vi "myRIO_BRig_RT__Case_Exp_State_initTrial_LC_ENL1__v3.vi"(6 "input_dataTrial":u16[][](array[numeric]), 7 "input_spout":enum16{"Left", "Right"}(ring), 8 "input_arrTrig":bool[](array[boolean]), 9 "input_dataBlock":u16[][](array[numeric]), 10 "input_dataLC":u16[](array[numeric]), 11 "input_dataCurrent":u16[](array[numeric])) -> (0 "output_arrTrig":bool[](array[boolean]), 4 "output_dataTrial":u16[][](array[numeric]), 5 "output_dataCurrent":u16[](array[numeric]))   [LabVIEW 2014]
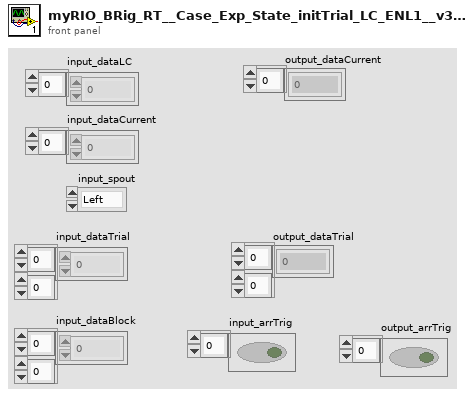
[diagram p1: front panel]
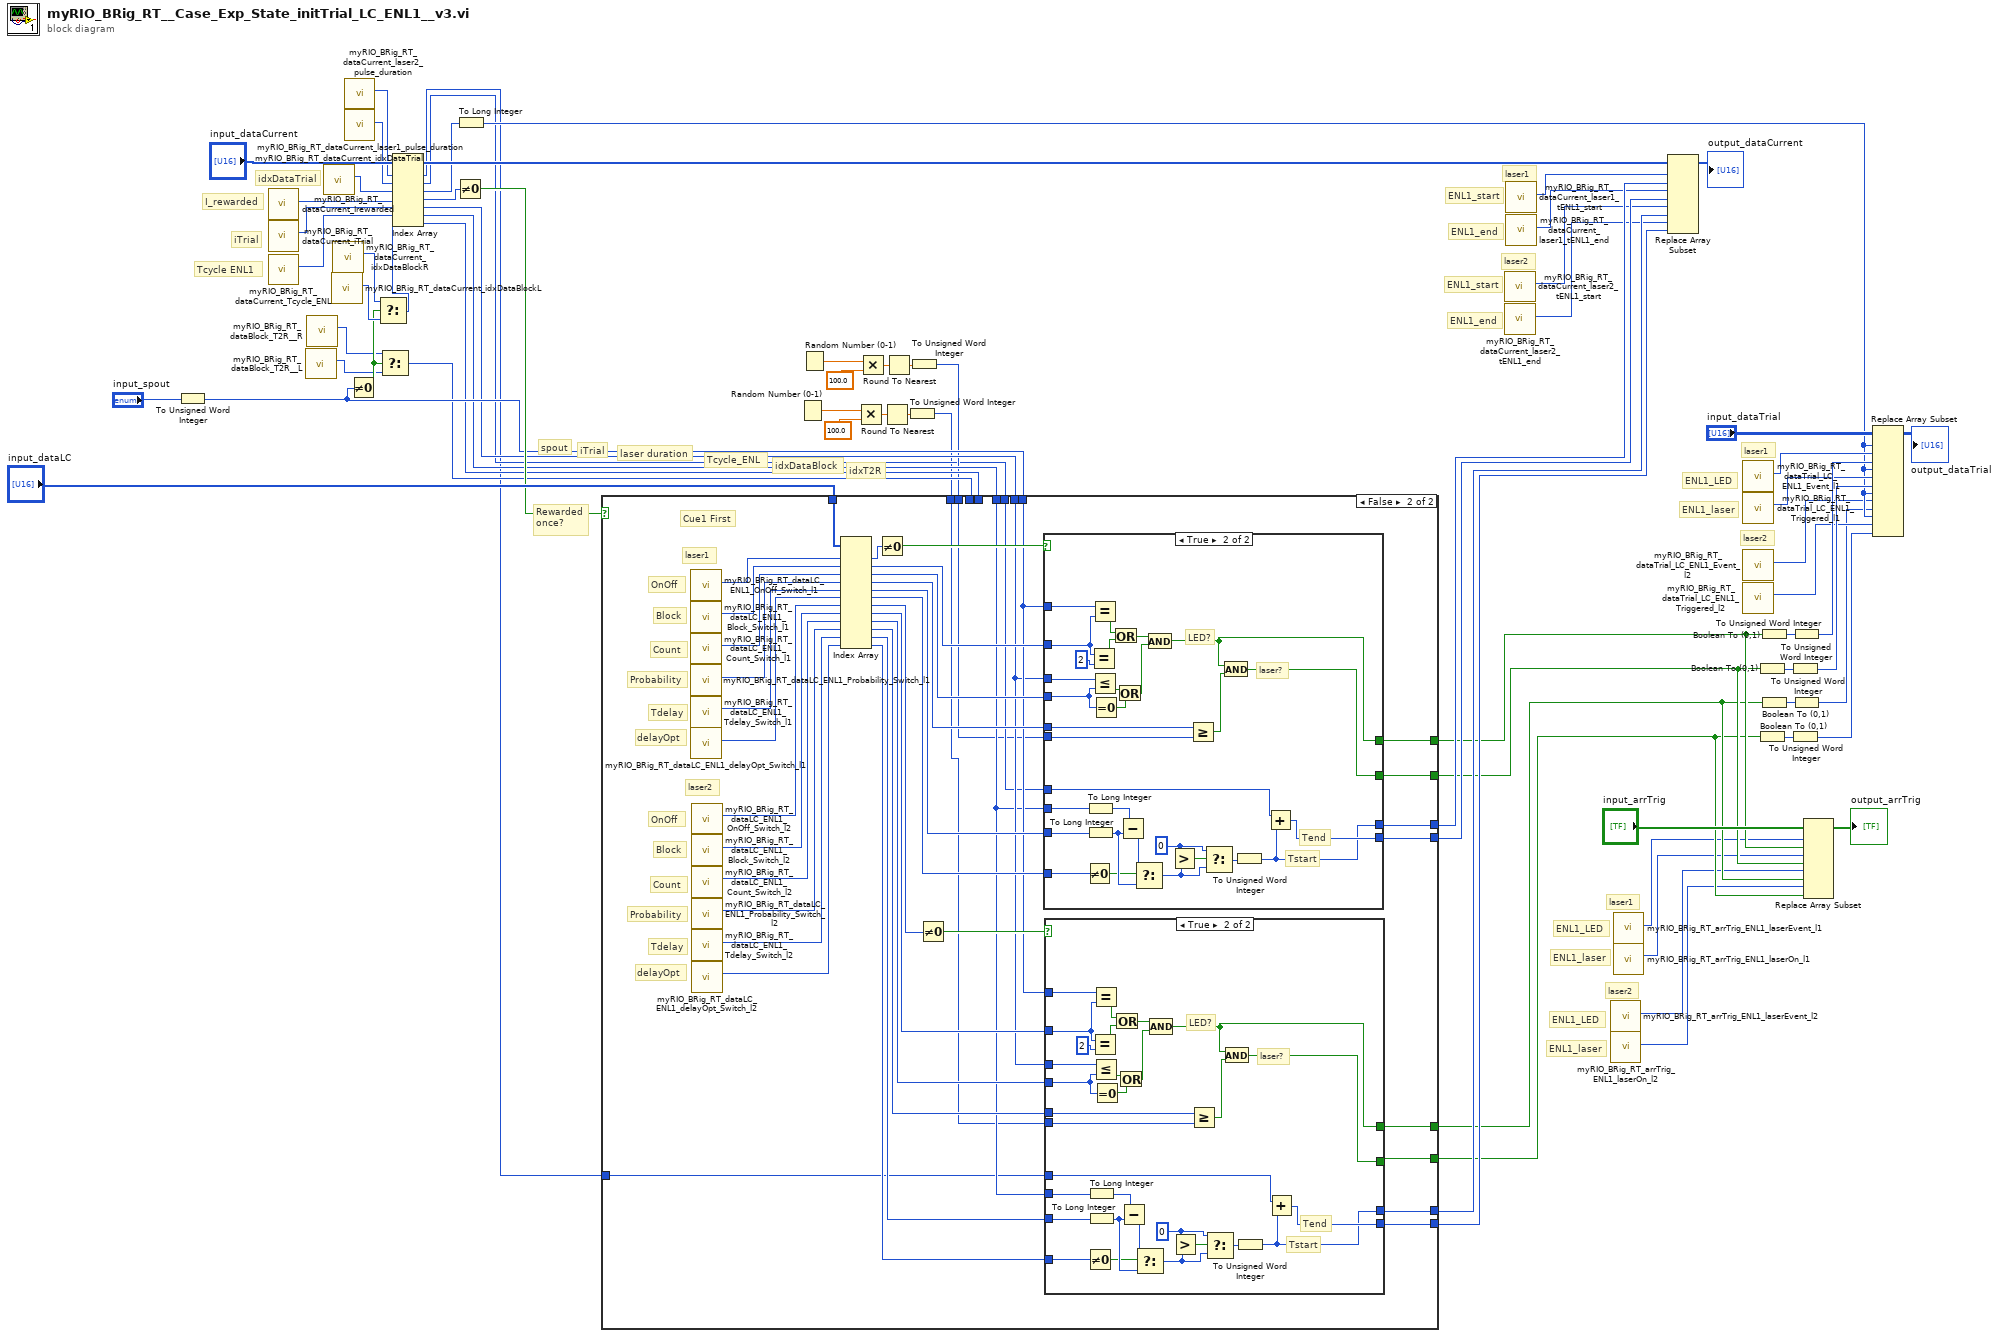
[diagram p0: block diagram]
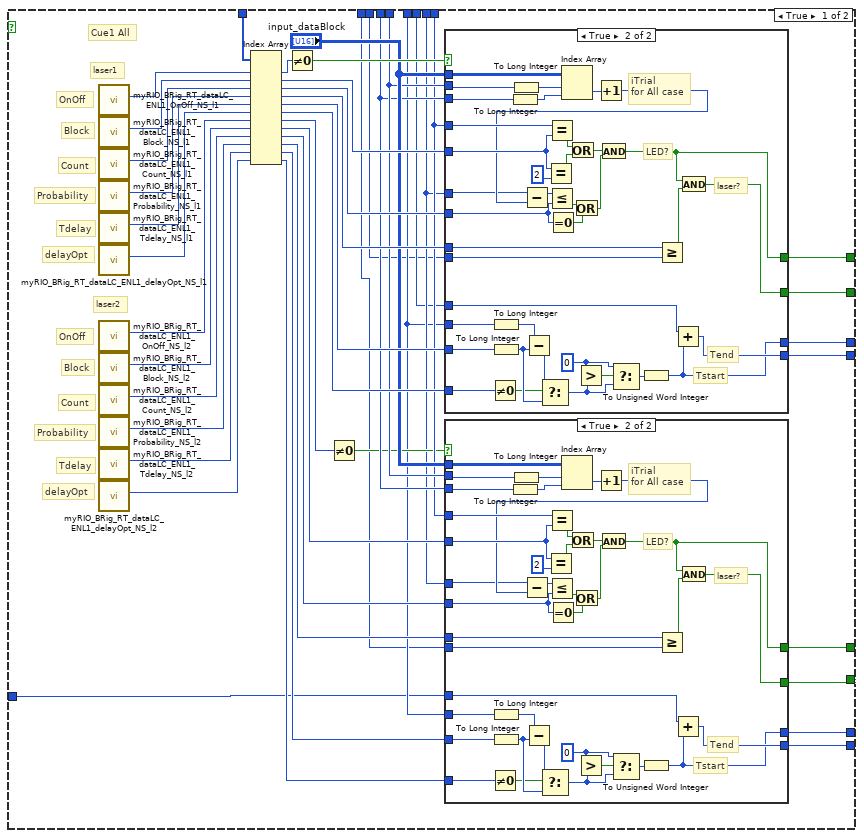
[diagram p2: hidden frame]
diagram:
  # "ENL1_LED"
  # "ENL1_laser"
  # "ENL1_end"
  # "ENL1_start"
  # "ENL1_end"
  # "ENL1_start"
  # "ENL1_LED"
  # "ENL1_laser"
  # "ENL1_LED"
  # "ENL1_laser"
  # "laser2"
  # "laser1"
  # "laser2"
  # "laser1"
  # "laser2"
  # "laser1"
  # "idxT2R"
  # "idxDataBlock"
  # "Tcycle_ENL"
  # "laser duration"
  # "iTrial"
  # "spout"
  # "Rewarded\nonce?"
  # "iTrial"
  # "idxDataTrial"
  # "Tcycle ENL1"
  # "I_rewarded"
  n1 = To Unsigned Word Integer(number="input_spout") -> (unsigned 16bit integer=w45:u16)
  n2 = call "myRIO_BRig_RT_dataCurrent_Irewarded.vi"() -> ("output_I_rewarded"=w67:i32)  [unwired: 11 in]
  n3 = call "myRIO_BRig_RT_dataCurrent_iTrial.vi"() -> ("output_iTrial"=w56:i32)  [unwired: 11 in]
  n4 = call "myRIO_BRig_RT_dataCurrent_Tcycle_ENL.vi"() -> ("output_ENL"=w25:i32)  [unwired: 11 in]
  n5 = call "myRIO_BRig_RT_dataBlock_T2R__L.vi"() -> ("output_T2R__L"=w50:i32)  [unwired: 11 in]
  n6 = call "myRIO_BRig_RT_dataBlock_T2R__R.vi"() -> ("output_T2R__R"=w51:i32)  [unwired: 11 in]
  n7 = call "myRIO_BRig_RT_dataCurrent_idxDataTrial.vi"() -> ("output_idxDataTrial"=w60:i32)  [unwired: 11 in]
  n8 = call "myRIO_BRig_RT_dataCurrent_idxDataBlockL.vi"() -> ("output_idxDataBlock__L"=w55:i32)  [unwired: 11 in]
  n9 = call "myRIO_BRig_RT_dataCurrent_idxDataBlockR.vi"() -> ("output_idxDataBlock__R"=w54:i32)  [unwired: 11 in]
  n10 = call "myRIO_BRig_RT_dataCurrent_laser2_pulse_duration.vi"() -> ("output_laser2_pulse_duration"=w9:i32)  [unwired: 11 in]
  n11 = call "myRIO_BRig_RT_dataCurrent_laser1_pulse_duration.vi"() -> ("output_laser1_pulse_duration"=w8:i32)  [unwired: 11 in]
  n12 = Not Equal To 0?(x=w45) -> (x != 0?=w52:bool)
  n13 = Select(t=w54, s=w52, f=w55) -> (s? t:f=w53:i32)
  n14 = Select(t=w51, s=w52, f=w50) -> (s? t:f=w41:i32)
  n15 = Index Array(array="input_dataCurrent", index #1=w9, index #2=w8, index #3=w60, index #4=w67, index #5=w56, index #6=w25, index #7=w53) -> (element #1=w6:u16, element #2=w7:u16, element #3=w59:u16, element #4=w68:u16, element #5=w44:u16, element #6=w43:u16, element #7=w42:u16)
  n16 = Not Equal To 0?(x=w68) -> (x != 0?=w46:bool)
  n17 = To Long Integer(number=w59) -> (32bit integer=w14:i32)
  n18 = Random Number (0-1)() -> (number: 0 to 1=w2:dbl)
  n19 = Random Number (0-1)() -> (number: 0 to 1=w37:dbl)
  n20 = Multiply(x=w2, y=100.0) -> (x*y=w3:dbl)
  n21 = Multiply(x=w37, y=100.0) -> (x*y=w38:dbl)
  n22 = Round To Nearest(number=w3) -> (nearest integer value=w4:dbl)
  n23 = Round To Nearest(number=w38) -> (nearest integer value=w39:dbl)
  n24 = To Unsigned Word Integer(number=w4) -> (unsigned 16bit integer=w1:u16)
  n25 = To Unsigned Word Integer(number=w39) -> (unsigned 16bit integer=w36:u16)
  n26 = case shown="False" w46 {
    tunnel: "input_dataLC" -> [w114 w232]
    tunnel: w45 -> [w103 w214]
    tunnel: w44 -> [w99 w212]
    tunnel: w7 -> [w96 w209]
    tunnel: w43 -> [w95 w208]
    tunnel: w42 -> [w105 _]
    tunnel: w41 -> [w104 _]
    tunnel: w36 -> [w70 w191]
    tunnel: [w92 w223] -> w29
    tunnel: [w91 w222] -> w28
    tunnel: [w90 w221] -> w35
    tunnel: [w89 w220] -> w34
    tunnel: [w88 w218] -> w27
    tunnel: [w87 w217] -> w26
    tunnel: [w86 w216] -> w33
    tunnel: [w85 w215] -> w32
    tunnel: w6 -> [w84 w205]
    tunnel: w1 -> [w71 w192]
    frame True {
      # "laser2"
      # "laser1"
      # "delayOpt"
      # "Count"
      # "Tdelay"
      # "Probability"
      # "OnOff"
      # "Block"
      # "delayOpt"
      # "Count"
      # "Tdelay"
      # "Probability"
      # "OnOff"
      # "Block"
      # "Cue1 All"
      n27 = call "myRIO_BRig_RT_dataLC_ENL1_OnOff_NS_l1.vi"() -> ("output_ENL1_OnOff_NS_l1"=w83:i32)  [unwired: 11 in]
      n28 = call "myRIO_BRig_RT_dataLC_ENL1_Block_NS_l1.vi"() -> ("output_ENL1_All_Block"=w82:i32)  [unwired: 11 in]
      n29 = call "myRIO_BRig_RT_dataLC_ENL1_Count_NS_l1.vi"() -> ("output_ENL1_Count_NS_l1"=w81:i32)  [unwired: 11 in]
      n30 = call "myRIO_BRig_RT_dataLC_ENL1_Probability_NS_l1.vi"() -> ("output_ENL1_Probability_NS_l1"=w80:i32)  [unwired: 11 in]
      n31 = call "myRIO_BRig_RT_dataLC_ENL1_Tdelay_NS_l1.vi"() -> ("output_ENL1_Tdelay_NS_l1"=w79:i32)  [unwired: 11 in]
      n32 = call "myRIO_BRig_RT_dataLC_ENL1_delayOpt_NS_l1.vi"() -> ("output_ENL1_delayOpt_NS_l1"=w78:i32)  [unwired: 11 in]
      n33 = call "myRIO_BRig_RT_dataLC_ENL1_OnOff_NS_l2.vi"() -> ("output_ENL1_OnOff_NS_l2"=w77:i32)  [unwired: 11 in]
      n34 = call "myRIO_BRig_RT_dataLC_ENL1_Block_NS_l2.vi"() -> ("output_ENL1_Block_NS_l2"=w76:i32)  [unwired: 11 in]
      n35 = call "myRIO_BRig_RT_dataLC_ENL1_Count_NS_l2.vi"() -> ("output_ENL1_Count_NS_l2"=w75:i32)  [unwired: 11 in]
      n36 = call "myRIO_BRig_RT_dataLC_ENL1_Probability_NS_l2.vi"() -> ("output_ENL1_Probability_NS_l2"=w74:i32)  [unwired: 11 in]
      n37 = call "myRIO_BRig_RT_dataLC_ENL1_Tdelay_NS_l2.vi"() -> ("output_ENL1_Tdelay_NS_l2"=w73:i32)  [unwired: 11 in]
      n38 = call "myRIO_BRig_RT_dataLC_ENL1_delayOpt_NS_l2.vi"() -> ("output_ENL1_delayOpt_NS_l2"=w72:i32)  [unwired: 11 in]
      n39 = Index Array(array=w114, index #1=w83, index #2=w82, index #3=w81, index #4=w80, index #5=w79, index #6=w78, index #7=w77, index #8=w76, index #9=w75, index #10=w74, index #11=w73, index #12=w72) -> (element #1=w109:u16, element #2=w107:u16, element #3=w113:u16, element #4=w112:u16, element #5=w111:u16, element #6=w110:u16, element #7=w102:u16, element #8=w100:u16, element #9=w98:u16, element #10=w97:u16, element #11=w94:u16, element #12=w93:u16)
      n40 = Not Equal To 0?(x=w109) -> (x != 0?=w108:bool)
      n41 = Not Equal To 0?(x=w102) -> (x != 0?=w101:bool)
      n42 = case shown="True" w108 {
        tunnel: w103 -> [_ w189]
        tunnel: w99 -> [_ w174]
        tunnel: [_ w169] -> w92
        tunnel: [_ w185] -> w91
        tunnel: [_ w160] -> w89
        tunnel: [_ w159] -> w90
        tunnel: w96 -> [_ w158]
        tunnel: w95 -> [_ w157]
        tunnel: w104 -> [_ w180]
        tunnel: w105 -> [_ w182]
        tunnel: w107 -> [_ w177]
        tunnel: w113 -> [_ w176]
        tunnel: w112 -> [_ w172]
        tunnel: w111 -> [_ w156]
        tunnel: w110 -> [_ w155]
        tunnel: "input_dataBlock" -> [_ w154]
        tunnel: w70 -> [_ w153]
        frame False {
        }
        frame True {
          w166 = 0 ("x")
          # "Tstart"
          # "Tend"
          # "iTrial\nfor All case"
          # "laser?"
          # "LED?"
          n43 = Not Equal To 0?(x=w155) -> (x != 0?=w163:bool)
          n44 = To Long Integer(number=w157) -> (32bit integer=w161:i32)
          n45 = To Long Integer(number=w156) -> (32bit integer=w164:i32)
          n46 = To Long Integer(number=w180) -> (32bit integer=w179:i32)
          n47 = To Long Integer(number=w182) -> (32bit integer=w181:i32)
          n48 = Subtract(x=w161, y=w164) -> (x-y=w162:i32)
          n49 = Select(t=w162, s=w163, f=w164) -> (s? t:f=w167:i32)
          n50 = Equal?(x=w177, y=u16 2) -> (x = y?=w187:bool)
          n51 = Equal?(x=w189, y=w177) -> (x = y?=w188:bool)
          n52 = Equal To 0?(x=w176) -> (x = 0?=w183:bool)
          n53 = Index Array(array=w154, index (row)=w181, index (col)=w179) -> (element=w178:u16)
          n54 = Or(x=w188, y=w187) -> (x .or. y?=w171:bool)
          n55 = Greater?(x=w166, y=w167) -> (0:w165:bool)
          n56 = Increment(x=w178) -> (x+1=w175:u16)
          n57 = Subtract(x=w174, y=w175) -> (x-y=w173:u16)
          n58 = Less Or Equal?(x=w173, y=w176) -> (x <= y?=w184:bool)
          n59 = Or(x=w184, y=w183) -> (x .or. y?=w170:bool)
          n60 = And(x=w171, y=w170) -> (x .and. y?=w169:bool)
          n61 = Select(t=w166, s=w165, f=w167) -> (s? t:f=w168:i32)
          n62 = To Unsigned Word Integer(number=w168) -> (unsigned 16bit integer=w159:u16)
          n63 = Greater Or Equal?(x=w172, y=w153) -> (x >= y?=w186:bool)
          n64 = Add(x=w158, y=w159) -> (x+y=w160:u16)
          n65 = And(x=w169, y=w186) -> (x .and. y?=w185:bool)
        }
      }
      n66 = case shown="True" w101 {
        tunnel: w103 -> [_ w151]
        tunnel: w99 -> [_ w136]
        tunnel: [_ w131] -> w88
        tunnel: [_ w147] -> w87
        tunnel: [_ w122] -> w85
        tunnel: [_ w121] -> w86
        tunnel: w84 -> [_ w120]
        tunnel: w95 -> [_ w119]
        tunnel: w104 -> [_ w142]
        tunnel: w105 -> [_ w144]
        tunnel: w100 -> [_ w139]
        tunnel: w98 -> [_ w138]
        tunnel: w97 -> [_ w134]
        tunnel: w94 -> [_ w118]
        tunnel: w93 -> [_ w117]
        tunnel: "input_dataBlock" -> [_ w116]
        tunnel: w71 -> [_ w115]
        frame False {
        }
        frame True {
          w128 = 0 ("x")
          # "Tstart"
          # "Tend"
          # "iTrial\nfor All case"
          # "laser?"
          # "LED?"
          n67 = Not Equal To 0?(x=w117) -> (x != 0?=w125:bool)
          n68 = To Long Integer(number=w119) -> (32bit integer=w123:i32)
          n69 = To Long Integer(number=w118) -> (32bit integer=w126:i32)
          n70 = To Long Integer(number=w142) -> (32bit integer=w141:i32)
          n71 = To Long Integer(number=w144) -> (32bit integer=w143:i32)
          n72 = Subtract(x=w123, y=w126) -> (x-y=w124:i32)
          n73 = Select(t=w124, s=w125, f=w126) -> (s? t:f=w129:i32)
          n74 = Equal?(x=w139, y=u16 2) -> (x = y?=w149:bool)
          n75 = Equal?(x=w151, y=w139) -> (x = y?=w150:bool)
          n76 = Equal To 0?(x=w138) -> (x = 0?=w145:bool)
          n77 = Index Array(array=w116, index (row)=w143, index (col)=w141) -> (element=w140:u16)
          n78 = Or(x=w150, y=w149) -> (x .or. y?=w133:bool)
          n79 = Greater?(x=w128, y=w129) -> (0:w127:bool)
          n80 = Increment(x=w140) -> (x+1=w137:u16)
          n81 = Subtract(x=w136, y=w137) -> (x-y=w135:u16)
          n82 = Less Or Equal?(x=w135, y=w138) -> (x <= y?=w146:bool)
          n83 = Or(x=w146, y=w145) -> (x .or. y?=w132:bool)
          n84 = And(x=w133, y=w132) -> (x .and. y?=w131:bool)
          n85 = Select(t=w128, s=w127, f=w129) -> (s? t:f=w130:i32)
          n86 = To Unsigned Word Integer(number=w130) -> (unsigned 16bit integer=w121:u16)
          n87 = Greater Or Equal?(x=w134, y=w115) -> (x >= y?=w148:bool)
          n88 = Add(x=w120, y=w121) -> (x+y=w122:u16)
          n89 = And(x=w131, y=w148) -> (x .and. y?=w147:bool)
        }
      }
    }
    frame False {
      # "laser2"
      # "laser1"
      # "delayOpt"
      # "Count"
      # "Tdelay"
      # "Probability"
      # "OnOff"
      # "Block"
      # "delayOpt"
      # "Count"
      # "Tdelay"
      # "Probability"
      # "OnOff"
      # "Block"
      # "Cue1 First"
      n90 = call "myRIO_BRig_RT_dataLC_ENL1_OnOff_Switch_l1.vi"() -> ("output_ENL1_OnOff_Switch_l1"=w204:i32)  [unwired: 11 in]
      n91 = call "myRIO_BRig_RT_dataLC_ENL1_Block_Switch_l1.vi"() -> ("output_ENL1_Block_Switch_l1"=w203:i32)  [unwired: 11 in]
      n92 = call "myRIO_BRig_RT_dataLC_ENL1_Count_Switch_l1.vi"() -> ("output_ENL1_Count_Switch_l1"=w202:i32)  [unwired: 11 in]
      n93 = call "myRIO_BRig_RT_dataLC_ENL1_Probability_Switch_l1.vi"() -> ("output_ENL1_Probability_Switch_l1"=w201:i32)  [unwired: 11 in]
      n94 = call "myRIO_BRig_RT_dataLC_ENL1_Tdelay_Switch_l1.vi"() -> ("output_ENL1_Tdelay_Switch_l1"=w200:i32)  [unwired: 11 in]
      n95 = call "myRIO_BRig_RT_dataLC_ENL1_delayOpt_Switch_l1.vi"() -> ("output_ENL1_delayOpt_Switch_l1"=w199:i32)  [unwired: 11 in]
      n96 = call "myRIO_BRig_RT_dataLC_ENL1_OnOff_Switch_l2.vi"() -> ("output_ENL1_OnOff_Switch_l2"=w198:i32)  [unwired: 11 in]
      n97 = call "myRIO_BRig_RT_dataLC_ENL1_Block_Switch_l2.vi"() -> ("output_ENL1_Block_Switch_l2"=w197:i32)  [unwired: 11 in]
      n98 = call "myRIO_BRig_RT_dataLC_ENL1_Count_Switch_l2.vi"() -> ("output_ENL1_Count_Switch_l2"=w196:i32)  [unwired: 11 in]
      n99 = call "myRIO_BRig_RT_dataLC_ENL1_Probability_Switch_l2.vi"() -> ("output_ENL1_Probability_Switch_l2"=w195:i32)  [unwired: 11 in]
      n100 = call "myRIO_BRig_RT_dataLC_ENL1_Tdelay_Switch_l2.vi"() -> ("output_ENL1_Tdelay_Switch_l2"=w194:i32)  [unwired: 11 in]
      n101 = call "myRIO_BRig_RT_dataLC_ENL1_delayOpt_Switch_l2.vi"() -> ("output_ENL1_delayOpt_Switch_l2"=w193:i32)  [unwired: 11 in]
      n102 = Index Array(array=w232, index #1=w204, index #2=w203, index #3=w202, index #4=w201, index #5=w200, index #6=w199, index #7=w198, index #8=w197, index #9=w196, index #10=w195, index #11=w194, index #12=w193) -> (element #1=w231:u16, element #2=w227:u16, element #3=w226:u16, element #4=w228:u16, element #5=w225:u16, element #6=w224:u16, element #7=w230:u16, element #8=w213:u16, element #9=w211:u16, element #10=w210:u16, element #11=w207:u16, element #12=w206:u16)
      n103 = Not Equal To 0?(x=w231) -> (x != 0?=w229:bool)
      n104 = Not Equal To 0?(x=w230) -> (x != 0?=w219:bool)
      n105 = case shown="True" w229 {
        tunnel: w214 -> [_ w291]
        tunnel: w227 -> [_ w290]
        tunnel: w212 -> [_ w289]
        tunnel: [_ w284] -> w223
        tunnel: [_ w283] -> w222
        tunnel: [_ w266] -> w220
        tunnel: w224 -> [_ w270]
        tunnel: w225 -> [_ w269]
        tunnel: [_ w265] -> w221
        tunnel: w226 -> [_ w282]
        tunnel: w208 -> [_ w268]
        tunnel: w209 -> [_ w267]
        tunnel: w191 -> [_ w264]
        tunnel: w228 -> [_ w263]
        frame False {
        }
        frame True {
          w276 = 0 ("x")
          # "Tstart"
          # "Tend"
          # "laser?"
          # "LED?"
          n106 = Not Equal To 0?(x=w270) -> (x != 0?=w273:bool)
          n107 = To Long Integer(number=w268) -> (32bit integer=w271:i32)
          n108 = To Long Integer(number=w269) -> (32bit integer=w274:i32)
          n109 = Equal?(x=w290, y=u16 2) -> (x = y?=w287:bool)
          n110 = Equal?(x=w291, y=w290) -> (x = y?=w288:bool)
          n111 = Less Or Equal?(x=w289, y=w282) -> (x <= y?=w281:bool)
          n112 = Equal To 0?(x=w282) -> (x = 0?=w280:bool)
          n113 = Or(x=w288, y=w287) -> (x .or. y?=w286:bool)
          n114 = Or(x=w281, y=w280) -> (x .or. y?=w279:bool)
          n115 = Subtract(x=w271, y=w274) -> (x-y=w272:i32)
          n116 = Select(t=w272, s=w273, f=w274) -> (s? t:f=w277:i32)
          n117 = Compound Arithmetic op=AND(w286, w279) -> (w284:bool)
          n118 = Greater?(x=w276, y=w277) -> (0:w275:bool)
          n119 = Greater Or Equal?(x=w263, y=w264) -> (x >= y?=w285:bool)
          n120 = Select(t=w276, s=w275, f=w277) -> (s? t:f=w278:i32)
          n121 = And(x=w284, y=w285) -> (x .and. y?=w283:bool)
          n122 = To Unsigned Word Integer(number=w278) -> (unsigned 16bit integer=w265:u16)
          n123 = Add(x=w267, y=w265) -> (x+y=w266:u16)
        }
      }
      n124 = case shown="True" w219 {
        tunnel: w214 -> [_ w261]
        tunnel: w213 -> [_ w260]
        tunnel: w212 -> [_ w259]
        tunnel: [_ w254] -> w218
        tunnel: [_ w253] -> w217
        tunnel: [_ w236] -> w215
        tunnel: w206 -> [_ w240]
        tunnel: w207 -> [_ w239]
        tunnel: [_ w235] -> w216
        tunnel: w211 -> [_ w252]
        tunnel: w208 -> [_ w238]
        tunnel: w205 -> [_ w237]
        tunnel: w192 -> [_ w234]
        tunnel: w210 -> [_ w233]
        frame False {
        }
        frame True {
          w246 = 0 ("x")
          # "Tstart"
          # "Tend"
          # "laser?"
          # "LED?"
          n125 = Not Equal To 0?(x=w240) -> (x != 0?=w243:bool)
          n126 = To Long Integer(number=w238) -> (32bit integer=w241:i32)
          n127 = To Long Integer(number=w239) -> (32bit integer=w244:i32)
          n128 = Equal?(x=w260, y=u16 2) -> (x = y?=w257:bool)
          n129 = Equal?(x=w261, y=w260) -> (x = y?=w258:bool)
          n130 = Less Or Equal?(x=w259, y=w252) -> (x <= y?=w251:bool)
          n131 = Equal To 0?(x=w252) -> (x = 0?=w250:bool)
          n132 = Or(x=w258, y=w257) -> (x .or. y?=w256:bool)
          n133 = Or(x=w251, y=w250) -> (x .or. y?=w249:bool)
          n134 = Subtract(x=w241, y=w244) -> (x-y=w242:i32)
          n135 = Select(t=w242, s=w243, f=w244) -> (s? t:f=w247:i32)
          n136 = Compound Arithmetic op=AND(w256, w249) -> (w254:bool)
          n137 = Greater?(x=w246, y=w247) -> (0:w245:bool)
          n138 = Greater Or Equal?(x=w233, y=w234) -> (x >= y?=w255:bool)
          n139 = Select(t=w246, s=w245, f=w247) -> (s? t:f=w248:i32)
          n140 = And(x=w254, y=w255) -> (x .and. y?=w253:bool)
          n141 = To Unsigned Word Integer(number=w248) -> (unsigned 16bit integer=w235:u16)
          n142 = Add(x=w237, y=w235) -> (x+y=w236:u16)
        }
      }
    }
  }
  n143 = call "myRIO_BRig_RT_dataCurrent_laser2_tENL1_start.vi"() -> ("output_laser2_tENL1_start"=w22:i32)  [unwired: 11 in]
  n144 = call "myRIO_BRig_RT_dataCurrent_laser2_tENL1_end.vi"() -> ("output_laser2_tENL1_end"=w21:i32)  [unwired: 11 in]
  n145 = call "myRIO_BRig_RT_dataCurrent_laser1_tENL1_start.vi"() -> ("output_laser1_tENL1_start"=w24:i32)  [unwired: 11 in]
  n146 = call "myRIO_BRig_RT_dataCurrent_laser1_tENL1_end.vi"() -> ("output_laser1_tENL1_end"=w23:i32)  [unwired: 11 in]
  n147 = call "myRIO_BRig_RT_arrTrig_ENL1_laserEvent_l2.vi"() -> ("output_arrTrig_ENL1_laserEvent_l2"=w16:i32)  [unwired: 11 in]
  n148 = call "myRIO_BRig_RT_arrTrig_ENL1_laserOn_l2.vi"() -> ("output_arrTrig_ENL1_laserOn_l2"=w15:i32)  [unwired: 11 in]
  n149 = call "myRIO_BRig_RT_arrTrig_ENL1_laserEvent_l1.vi"() -> ("output_arrTrig_ENL1_laserEvent_l1"=w18:i32)  [unwired: 11 in]
  n150 = call "myRIO_BRig_RT_arrTrig_ENL1_laserOn_l1.vi"() -> ("output_arrTrig_ENL1_laserOn_l1"=w17:i32)  [unwired: 11 in]
  n151 = Replace Array Subset(array="input_dataCurrent", new element #1=w35, index #1=w24, new element #2=w34, index #2=w23, new element #3=w33, index #3=w22, new element #4=w32, index #4=w21) -> (→"output_dataCurrent":u16[])
  n152 = call "myRIO_BRig_RT_dataTrial_LC_ENL1_Event_l1.vi"() -> ("output_LC_ENL1_Event_l1"=w20:i32)  [unwired: 11 in]
  n153 = call "myRIO_BRig_RT_dataTrial_LC_ENL1_Triggered_l1.vi"() -> ("output_LC_ENL1_Triggered_l1"=w19:i32)  [unwired: 11 in]
  n154 = call "myRIO_BRig_RT_dataTrial_LC_ENL1_Event_l2.vi"() -> ("output_LC_ENL1_Event_l2"=w13:i32)  [unwired: 11 in]
  n155 = call "myRIO_BRig_RT_dataTrial_LC_ENL1_Triggered_l2.vi"() -> ("output_LC_ENL1_Triggered_l2"=w12:i32)  [unwired: 11 in]
  n156 = Boolean To (0,1)(Boolean=w28) -> (0, 1=w63:i16)
  n157 = Boolean To (0,1)(Boolean=w26) -> (0, 1=w31:i16)
  n158 = Boolean To (0,1)(Boolean=w29) -> (0, 1=w64:i16)
  n159 = Boolean To (0,1)(Boolean=w27) -> (0, 1=w30:i16)
  n160 = To Unsigned Word Integer(number=w63) -> (unsigned 16bit integer=w57:u16)
  n161 = To Unsigned Word Integer(number=w31) -> (unsigned 16bit integer=w10:u16)
  n162 = To Unsigned Word Integer(number=w64) -> (unsigned 16bit integer=w58:u16)
  n163 = To Unsigned Word Integer(number=w30) -> (unsigned 16bit integer=w11:u16)
  n164 = Replace Array Subset(array="input_arrTrig", new element #1=w29, index #1=w18, new element #2=w28, index #2=w17, new element #3=w27, index #3=w16, new element #4=w26, index #4=w15) -> (→"output_arrTrig":bool[])
  n165 = Replace Array Subset(array="input_dataTrial", new element #1=w58, index (row) #1=w14, index (col) #1=w20, new element #2=w57, index (row) #2=w14, index (col) #2=w19, new element #3=w11, index (row) #3=w14, index (col) #3=w13, new element #4=w10, index (row) #4=w14, index (col) #4=w12) -> (→"output_dataTrial":u16[][])
